vi "New PID Move Talon (1).vi"(8 "Cluster 3":T2={"Left Encoder"="Talon1", "Right Encoder"="Talon4", "Gyro Refnum"="Gyro", "Device Number"=enum."Dev0", "Right Refnum"="Talon5", "Left Refnum"="Talon2", "Right Intake"="Talon9", "Left Intake"="Talon7"}, 9 "Timeout":i16, 10 "Target Distance":dbl format="%#_13g", 11 "Target Angle":dbl) -> (0 "Cluster 2":T2={"Left Encoder"="Talon1", "Right Encoder"="Talon4", "Gyro Refnum"="Gyro", "Device Number"=enum."Dev0", "Right Refnum"="Talon5", "Left Refnum"="Talon2", "Right Intake"="Talon9", "Left Intake"="Talon7"})   [LabVIEW 2017]
uses:
  <vilib>/Rock Robotics/WPI/ThirdParty/Sensors/navX/_TypeDefs/FRIC_navX_DeviceNumbersTypeDef.ctl
  Public/Documents/Cross The Road Electronics/Phoenix-LabVIEW/Motor Controller/Controls/CTRE_Phoenix_MotorControl_ControlMode.ctl
  <vilib>/Rock Robotics/WPI/ThirdParty/Phoenix-LabVIEW/Motor Controller/Get/CTRE_Phoenix_MotorController_GetQuadratureData.vi
  <vilib>/addons/control/pid/pid.llb/PID (DBL).vi
  <vilib>/addons/control/pid/NI_PID_pid.lvlib
panel:
  out "In Range":dbl
  out "A-Setpoint":dbl
  in  "D - Lower Limit":dbl=-0.6 format="%#_13g"
  in  "D - Upper Limit":dbl=0.6 format="%#_13g"
  in  "A - Lower Limit":dbl=-1.0 format="%#_13g"
  in  "A - Upper Limit":dbl=1.0 format="%#_13g"
  out "D - Low Threshold":dbl
  out "D - High Threshold":dbl
  out "Cluster":cluster{dbl, dbl}
  out "Angle Modifier":dbl format="%.2f"
  out "Distance Modifier":dbl format="%.2f"
  out "Quadrature Position 4":i32
  out "Quadrature Position 1":i32
  out "Elapsed Time":u32
  out "Distance":i32
  out "Angle":dbl
  in  "A-D":dbl=0.001 format="%#_13g"
  in  "A-I":dbl format="%#_13g"
  in  "A-P":dbl=0.065 format="%#_13g"
  out "Right":dbl
  out "Left":dbl
  in  "D-P":dbl=5e-05 format="%#_13g"
  in  "D-I":dbl format="%#_13g"
  in  "D-D":dbl=1e-07 format="%#_13g"
  out "error out":errorcluster
  in  "error in":errorcluster
  # "pos 1-pos8=distance"
  # "5e-5\n0\n1e-7"
  # ".065\n0\n.001"
  # "Miami Valley\nDistance\n3E-5\n0\n.001\n.7\n-.7\n\nAngle\n.075\n0\n0\n.5\n-.5\n\n25k=20\" 20.25\"\n50k=39.75\"\n100k=78.5\"\n150k=116.5"
  # ".0002"
  # "4"
  # "2.5E-5"
  # "ALPHA encoders\nTalon1\nTalon4\n\nALPHA drive\nTalon2\nTalon5"
  # ".00001"
  # ".0005"
  # "8e-5/0/1e-7"
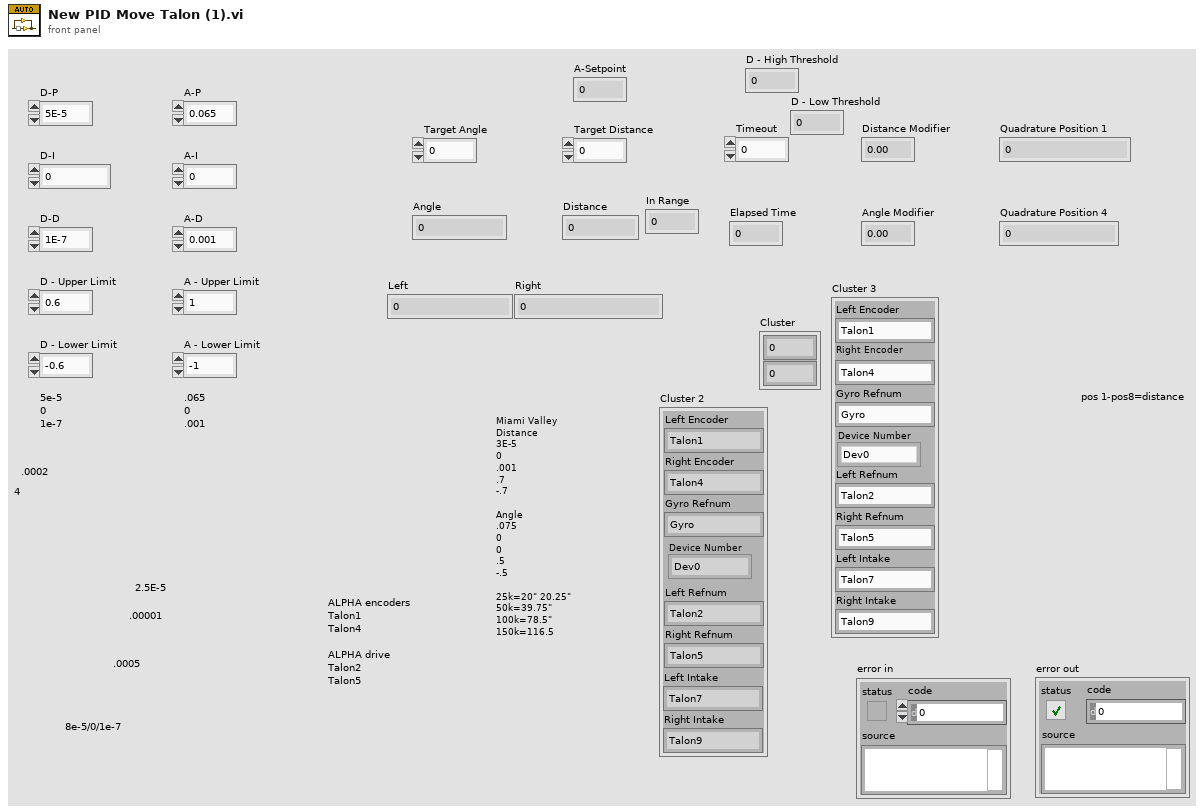
[diagram p1: front panel]
types:
  T1 = typedef "FRIC_navX_DeviceNumbersTypeDef.ctl" = enum16{"Dev0", "Dev1", "Dev2", "Dev3"}
  T2 = cluster{"Left Encoder":string, "Right Encoder":string, "Gyro Refnum":string, "Device Number":T1, "Right Refnum":string, "Left Refnum":string, "Right Intake":string, "Left Intake":string}
  T3 = typedef "CTRE_Phoenix_MotorControl_ControlMode.ctl" = u16
  T4 = typedef "WPI_GyroDevRef.ctl" = cluster{"DevStatus":errorcluster, "Analog Channel":T5, "Gain (VoltsPerDegree/Second)":dbl, "Gyro Type":enum16{"Analog", "XRS450"}, "Handle":i32, "SPI Bus":T6, "Device Found":bool, "Sample Rate":dbl, "Calibrate On Open":bool, "Offset":dbl}
  T5 = typedef "FPGA_AIChannel.ctl" = enum8{"AI 0", "AI 1", "AI 2", "AI 3", "AI MXP 0", "AI MXP 1", "AI MXP 2", "AI MXP 3", "Invalid"}
  T6 = typedef "spi_bus.ctl" = enum16{"SPI On-Board, CS0", "SPI On-Board, CS1", "SPI On-Board, CS2", "SPI On-Board, CS3", "SPI MXP", "Invalid"}
  T7 = typedef "WPI_MotorControlDeviceRef.ctl" = cluster{"DeviceStatus":errorcluster, "Type":T8, "PWM":cluster{"PWM Channel":T9, "DeadBand":T10}, "CAN":cluster{"Device Number":u8, "SetOutput VI Ref":variant, "GetOutput VI Ref":variant, "Enable VI Ref":variant, "Disable VI Ref":variant, "Data":variant}, "Invert":bool, "DIO PWM":cluster{"PWM \"Enable\" Channel":T9, "DIOChannel":T11, "PWM Rate":dbl}}
  T8 = typedef "WPI_MotorControlType.ctl" = enum16{"PWM", "CAN", "DIO PWM"}
  T9 = typedef "FPGA_DIOPWMChannel.ctl" = enum8{"PWM 0", "PWM 1", "PWM 2", "PWM 3", "PWM 4", "PWM 5", "PWM 6", "PWM 7", "PWM 8", "PWM 9", "PWM MXP 0", "PWM MXP 1", "PWM MXP 2", "PWM MXP 3", "PWM MXP 4", "PWM MXP 5", "PWM MXP 6", "PWM MXP 7", "PWM MXP 8", "PWM MXP 9", "Invalid"}
  T10 = typedef "WPI_PWMDeadband.ctl" = cluster{"Name":string, "maxPositivePwm":i32, "minPositivePwm":i32, "centerPwm":i32, "maxNegativePwm":i32, "minNegativePwm":i32, "angularRange":u16}
  T11 = typedef "FPGA_DIOChannel.ctl" = enum8{"DIO 0", "DIO 1", "DIO 2", "DIO 3", "DIO 4", "DIO 5", "DIO 6", "DIO 7", "DIO 8", "DIO 9", "DIO MXP 0", "DIO MXP 1", "DIO MXP 2", "DIO MXP 3", "DIO MXP 4", "DIO MXP 5", "DIO MXP 6", "DIO MXP 7", "DIO MXP 8", "DIO MXP 9", "DIO MXP 10", "DIO MXP 11", "DIO MXP 12", "DIO MXP 13", "DIO MXP 14", "DIO MXP 15", "SPI Port CS1", "SPI Port CS2", "SPI Port CS3", "SPI Port MISO", "SPI Port MOSI", "Invalid"}
  T12 = cluster{"D - Upper Limit":dbl, "D - Lower Limit":dbl}
  T13 = cluster{"A - Upper Limit":dbl, "A - Lower Limit":dbl}
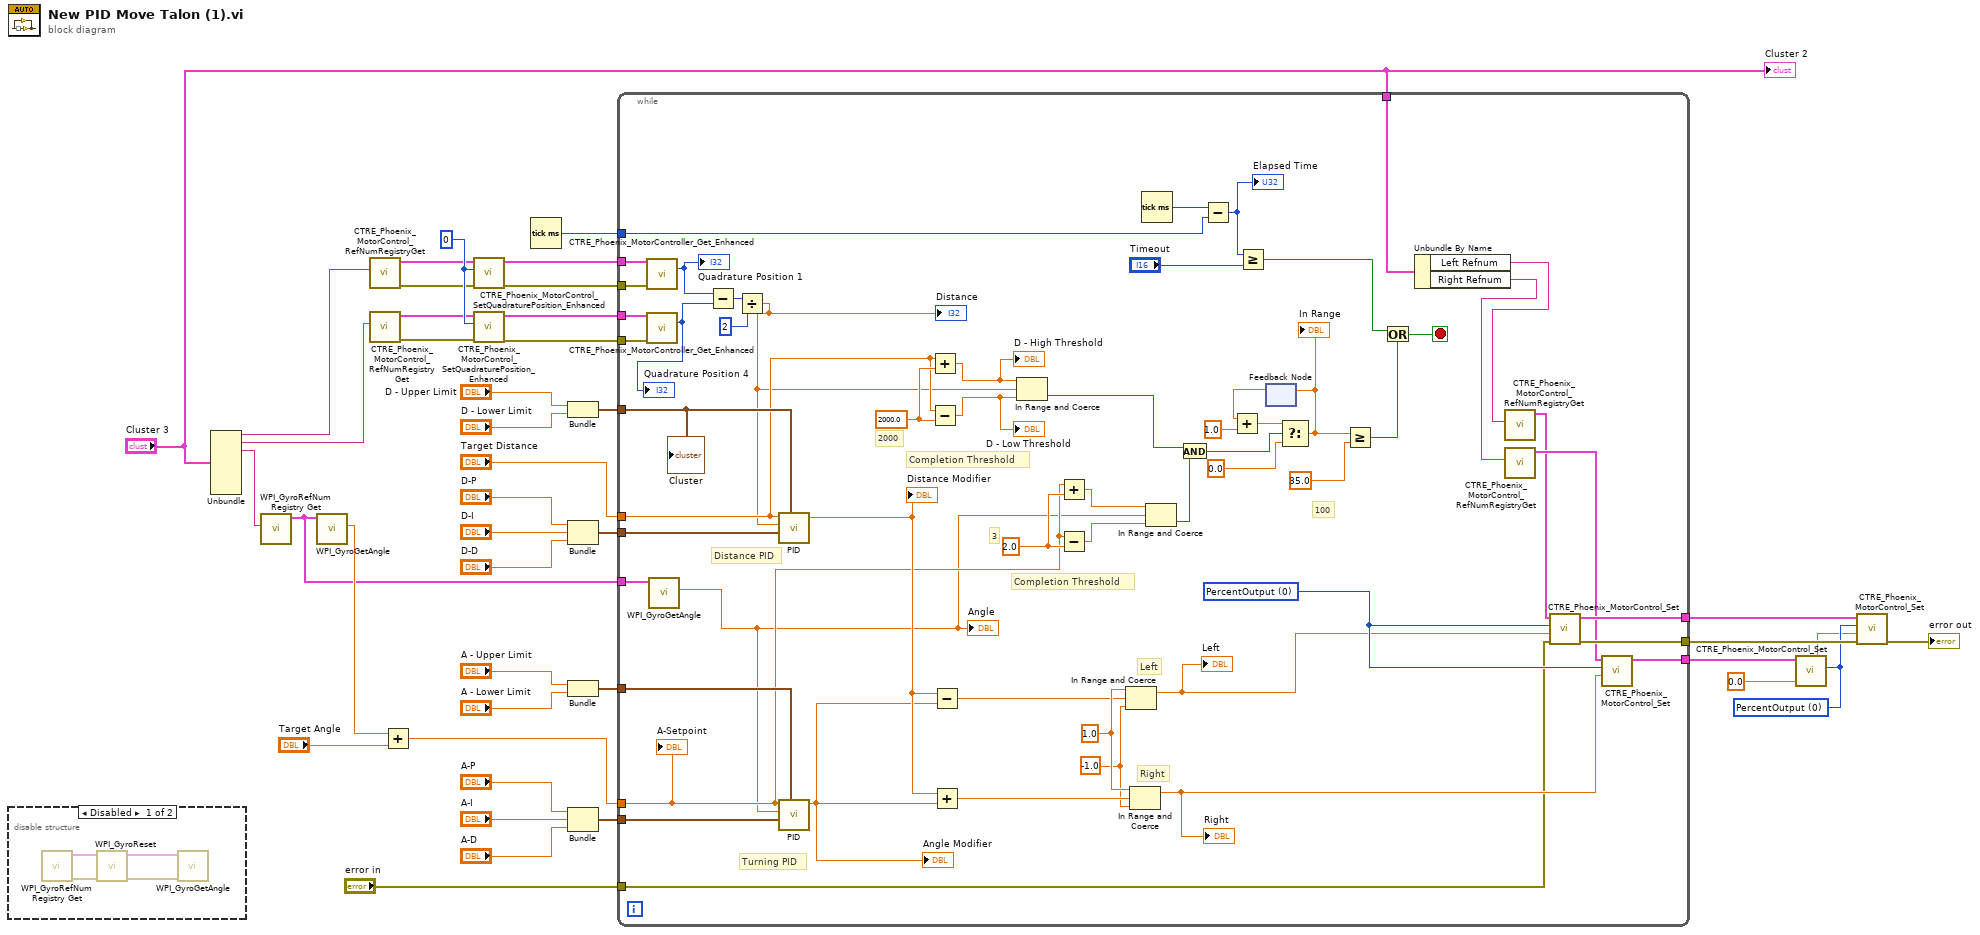
[diagram p0: block diagram]
diagram:
  w3 = 0.0 ("Output")
  w4 = T3 0 items=["PercentOutput"=0, "Position"=1, "Velocity"=2, "Current"=3, "Follower"=5, "MotionProfile"=6, "MotionMagic"=7, "MotionMagicArc"=8, "MotionProfileArc"=10, "Disabled"=15] ("Control Mode")
  w23 = 0 ("New Position")
  n1 = disable-structure shown="Disabled" {
    frame Disabled {
      n2 = call <vilib>:"WPI_GyroRefNum Registry Get.vi"() -> ("error out"=w43:errorcluster, "GyroDevRef"=w44:T4)  [unwired: 10 in]
      n3 = call <vilib>:"WPI_GyroReset.vi"("error in"=w43, "GyroDevRef"=w44) -> ("error out"=w41:errorcluster, "GyroDevRef"=w42:T4)  [unwired: 8 in]
      n4 = call <vilib>:"WPI_GyroGetAngle.vi"("error in"=w41, "GyroDevRef"=w42) -> ()  [unwired: 5 in, 5 out]
    }
    frame Enabled {
    }
  }
  n5 = Unbundle("Cluster 3") -> ("Left Encoder"=w17:string, "Right Encoder"=w16:string, "Gyro Refnum"=w13:string)  [unwired: 5 out]
  n6 = call <vilib>:"WPI_GyroRefNum Registry Get.vi"("refnum name"=w13) -> ("GyroDevRef"=w11:T4)  [unwired: 9 in, 1 out]
  n7 = call <vilib>:"WPI_GyroGetAngle.vi"("GyroDevRef"=w11) -> ("Angle"=w12:dbl)  [unwired: 6 in, 4 out]
  n8 = call <vilib>:"CTRE_Phoenix_MotorControl_RefNumRegistryGet.vi"("refnum name"=w17) -> ("error out"=w19:errorcluster, "PhoenixMotorControlDevRef"=w10:T7)  [unwired: 9 in]
  n9 = call <vilib>:"CTRE_Phoenix_MotorControl_RefNumRegistryGet.vi"("refnum name"=w16) -> ("error out"=w21:errorcluster, "PhoenixMotorControlDevRef"=w9:T7)  [unwired: 9 in]
  n10 = Add(x=w12, y="Target Angle") -> (x+y=w14:dbl)
  n11 = call "CTRE_Phoenix_MotorControl_SetQuadraturePosition_Enhanced.vi"("error in (no error)"=w19, "New Position"=w23, "PhoenixMotorControlDevRef"=w10) -> ("error out"=w20:errorcluster, "PhoenixMotorControlDevRef"=w25:T7)  [unwired: 7 in]
  n12 = call "CTRE_Phoenix_MotorControl_SetQuadraturePosition_Enhanced.vi"("error in (no error)"=w21, "New Position"=w23, "PhoenixMotorControlDevRef"=w9) -> ("error out"=w22:errorcluster, "PhoenixMotorControlDevRef"=w24:T7)  [unwired: 7 in]
  n13 = Tick Count (ms)() -> (millisecond timer value=w18:u32)
  n14 = Bundle("D - Upper Limit"="D - Upper Limit", "D - Lower Limit"="D - Lower Limit") -> (w38:T12)  [unwired: 1 in]
  n15 = Bundle("D-P"="D-P", "D-I"="D-I", "D-D"="D-D") -> (w27:cluster{"D-P":dbl, "D-I":dbl, "D-D":dbl})  [unwired: 1 in]
  n16 = Bundle("A - Upper Limit"="A - Upper Limit", "A - Lower Limit"="A - Lower Limit") -> (w35:T13)  [unwired: 1 in]
  n17 = Bundle("A-P"="A-P", "A-I"="A-I", "A-D"="A-D") -> (w31:cluster{"A-P":dbl, "A-I":dbl, "A-D":dbl})  [unwired: 1 in]
  n18 = while {
    tunnel: w38 -> [w101]
    tunnel: w35 -> [w99]
    tunnel: w31 -> [w95]
    tunnel: w27 -> [w94]
    tunnel: "Target Distance" -> [w82]
    tunnel: w14 -> [w75]
    tunnel: w24 -> [w92]
    tunnel: w25 -> [w91]
    tunnel: w22 -> [w90]
    tunnel: w20 -> [w89]
    tunnel: w18 -> [w86]
    tunnel: w11 -> [w65]
    tunnel: [w60] -> w8
    tunnel: [w59] -> w6
    tunnel: [w58] -> w5
    tunnel: "Cluster 3" -> [w57]
    tunnel: "error in" -> [w48]
    stop <- w70 stop-if-true
    w49 = -1.0
    w63 = T3 0 items=["PercentOutput"=0, "Position"=1, "Velocity"=2, "Current"=3, "Follower"=5, "MotionProfile"=6, "MotionMagic"=7, "MotionMagicArc"=8, "MotionProfileArc"=10, "Disabled"=15] ("Control Mode")
    w76 = 2.0
    w93 = 2000.0
    w100 = 1.0
    # "100"
    # "3"
    # "2000"
    # "Completion Threshold"
    # "Completion Threshold"
    # "Right"
    # "Left"
    # "Turning PID"
    # "Distance PID"
    n19 = call-poly <vilib>:"CTRE_Phoenix_MotorController_Get_Enhanced.vi"("PhoenixMotorControlDevRef"=w91, "error in"=w89) -> ("Quadrature Position"=w45:i32)  [unwired: 10 in, 3 out]
    "Quadrature Position 1" <- w45
    n20 = call-poly <vilib>:"CTRE_Phoenix_MotorController_Get_Enhanced.vi"("PhoenixMotorControlDevRef"=w92, "error in"=w90) -> ("Quadrature Position"=w46:i32)  [unwired: 10 in, 3 out]
    "Quadrature Position 4" <- w46
    n21 = call <vilib>:"WPI_GyroGetAngle.vi"("GyroDevRef"=w65) -> ("Angle"=w64:dbl)  [unwired: 6 in, 4 out]
    "Angle" <- w64
    n22 = Subtract(x=w45, y=w46) -> (x-y=w67:i32)
    n23 = Divide(x=w67, y=2) -> (x/y=w47:dbl)
    "Distance" <- w47
    n24 = call-poly <vilib>:"PID.vi"("output range"=w101, "PID gains"=w94, "process variable"=w47, "setpoint"=w82) -> ("output"=w98:dbl)  [unwired: 6 in, 1 out]
    "Distance Modifier" <- w98
    n25 = call-poly <vilib>:"PID.vi"("output range"=w99, "PID gains"=w95, "process variable"=w64, "setpoint"=w75) -> ("output"=w69:dbl)  [unwired: 6 in, 1 out]
    "Angle Modifier" <- w69
    n26 = Add(x=w82, y=w93) -> (x+y=w81:dbl)
    "D - High Threshold" <- w81
    n27 = Subtract(x=w82, y=w93) -> (x-y=w80:dbl)
    "D - Low Threshold" <- w80
    n28 = Subtract(x=w98, y=w69) -> (x-y=w96:dbl)
    n29 = Add(x=w98, y=w69) -> (x+y=w97:dbl)
    n30 = In Range and Coerce(upper limit=w81, x=w47, lower limit=w80) -> (In Range?=w79:bool)  [unwired: 1 out]
    n31 = Add(x=w75, y=w76) -> (x+y=w77:dbl)
    n32 = Subtract(x=w75, y=w76) -> (x-y=w78:dbl)
    n33 = In Range and Coerce(upper limit=w100, x=w96, lower limit=w49) -> (coerced(x)=w62:dbl)  [unwired: 1 out]
    "Left" <- w62
    n34 = In Range and Coerce(upper limit=w100, x=w97, lower limit=w49) -> (coerced(x)=w61:dbl)  [unwired: 1 out]
    "Right" <- w61
    n35 = Tick Count (ms)() -> (millisecond timer value=w88:u32)
    n36 = In Range and Coerce(upper limit=w77, x=w64, lower limit=w78) -> (In Range?=w74:bool)  [unwired: 1 out]
    n37 = And(x=w79, y=w74) -> (x .and. y?=w73:bool)
    n38 = Subtract(x=w88, y=w86) -> (x-y=w87:u32)
    "Elapsed Time" <- w87
    n39 = Greater Or Equal?(x=w87, y="Timeout") -> (x >= y?=w72:bool)
    n40 = feedback #1() -> (w84:dbl)  [unwired: 1 in]
    n41 = Add(x=w84, y=1.0) -> (x+y=w85:dbl)
    n42 = Select(t=w85, s=w73, f=0.0) -> (s? t:f=w83:dbl)
    "In Range" <- w83
    n43 = feedback-in #1(w83) -> ()
    n44 = Greater Or Equal?(x=w83, y=35.0) -> (x >= y?=w71:bool)
    n45 = Or(x=w72, y=w71) -> (x .or. y?=w70:bool)
    n46 = Unbundle By Name(w57) -> ("Left Refnum"=w56:string, "Right Refnum"=w55:string)
    n47 = call <vilib>:"CTRE_Phoenix_MotorControl_RefNumRegistryGet.vi"("refnum name"=w56) -> ("PhoenixMotorControlDevRef"=w53:T7)  [unwired: 9 in, 1 out]
    n48 = call <vilib>:"CTRE_Phoenix_MotorControl_RefNumRegistryGet.vi"("refnum name"=w55) -> ("PhoenixMotorControlDevRef"=w54:T7)  [unwired: 9 in, 1 out]
    n49 = call <vilib>:"CTRE_Phoenix_MotorControl_Set.vi"("error in (no error)"=w48, "Output"=w62, "Control Mode"=w63, "PhoenixMotorControlDevRef"=w53) -> ("error out"=w60:errorcluster, "PhoenixMotorControlDevRef"=w59:T7)  [unwired: 6 in]
    n50 = call <vilib>:"CTRE_Phoenix_MotorControl_Set.vi"("Output"=w61, "Control Mode"=w63, "PhoenixMotorControlDevRef"=w54) -> ("PhoenixMotorControlDevRef"=w58:T7)  [unwired: 7 in, 1 out]
    "Cluster" <- w101
    "A-Setpoint" <- w75
  }
  n51 = call <vilib>:"CTRE_Phoenix_MotorControl_Set.vi"("Output"=w3, "Control Mode"=w4, "PhoenixMotorControlDevRef"=w5) -> ()  [unwired: 7 in, 2 out]
  n52 = call <vilib>:"CTRE_Phoenix_MotorControl_Set.vi"("error in (no error)"=w8, "Output"=w3, "Control Mode"=w4, "PhoenixMotorControlDevRef"=w6) -> ("error out"=→"error out":errorcluster)  [unwired: 6 in, 1 out]
  "Cluster 2" <- "Cluster 3"
